vi "OnOff Read.vi"(8 "error in":errorcluster, 11 "Power Supply In":refnum<class "Power Supply.lvclass">) -> (0 "error out":errorcluster, 1 "Changed or First Call?":bool, 2 "OnOff Out":bool, 3 "Power Supply Out":refnum<class "Power Supply.lvclass">)   [LabVIEW 2023, in "Power Supply.lvclass"]
uses:
  Power Supply.lvclass
  Power Supply.lvclass/Power Supply.ctl
  Low Level Capabilities/OnOff/OnOff.lvclass
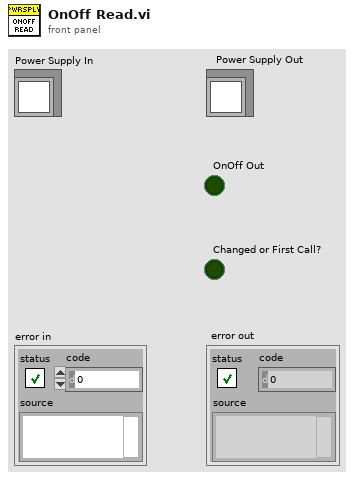
[diagram p1: front panel]
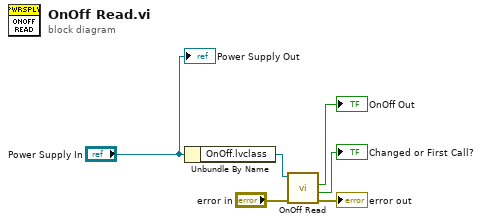
[diagram p0: block diagram]
diagram:
  n1 = Unbundle By Name("Power Supply In") -> ("OnOff.lvclass"=w5:refnum<class "OnOff.lvclass">)
  n2 = call-dynamic "OnOff Read.vi"("error in"="error in", "OnOff in"=w5) -> ("error out"=→"error out":errorcluster, "Changed or First Call?"=→"Changed or First Call?":bool, "OnOff ACT"=→"OnOff Out":bool)  [unwired: 6 in, 1 out]
  "Power Supply Out" <- "Power Supply In"
